vi "H5D Create 1D array.vi"(5 "chunk size":u32=16250, 6 "compress level":i32=9, 7 "compress?":bool, 8 "error in (no error)":errorcluster, 9 "defined type":i32(ring)=17 items=["None", "IEEE_F32BE", "IEEE_F32LE", "IEEE_F64BE", "IEEE_F64LE", "NATIVE_CHAR", "NATIVE_SCHAR", "NATIVE_UCHAR", "NATIVE_SHORT", "NATIVE_USHORT", "NATIVE_INT", "NATIVE_UINT", "NATIVE_LONG", "NATIVE_ULONG", "NATIVE_LLONG", "NATIVE_ULLONG", "NATIVE_FLOAT", "NATIVE_DOUBLE", "NATIVE_LDOUBLE", "NATIVE_B8", "NATIVE_B16", "NATIVE_B32", "NATIVE_B64", "NATIVE_OPAQUE", "NATIVE_HADDR", "NATIVE_HSIZE", "NATIVE_HSSIZE", "NATIVE_HERR", "NATIVE_HBOOL", "STD_U8LE", "STD_U8BE", "STD_U16LE", "STD_U16BE", "STD_U32LE", "STD_U32BE", "STD_U64LE", "STD_U64BE", "STD_B8LE", "STD_B8BE", "STD_B16LE", "STD_B16BE", "STD_B32LE", "STD_B32BE", "STD_B64LE", "STD_B64BE", "STD_REF_OBJ", "STD_REF_DSETREG", "C_S1", "STD_I8LE", "STD_I8BE", "STD_I16LE", "STD_I16BE", "STD_I32LE", "STD_I32BE", "STD_I64LE", "STD_I64BE", ""], 10 "name":string, 11 "loc_id":i32) -> (0 "error out":errorcluster, 1 "space_id":i32, 2 "plist out":i32, 3 "dataset_id":i32)   [LabVIEW 2011]
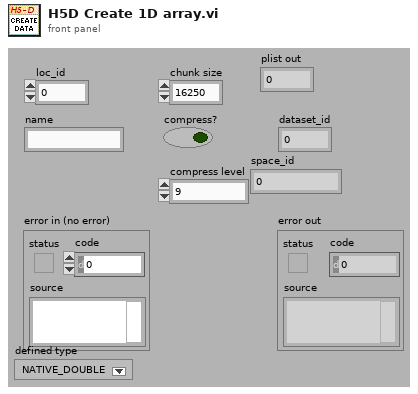
[diagram p1: front panel]
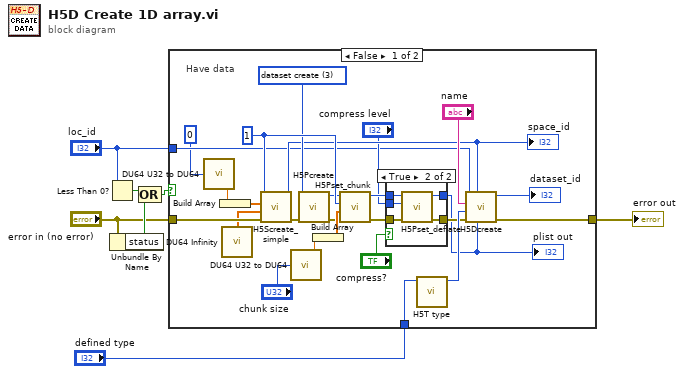
[diagram p0: block diagram]
diagram:
  n1 = Less Than 0?(x="loc_id") -> (x < 0?=w5:bool)
  n2 = Unbundle By Name("error in (no error)") -> ("status"=w6:bool)
  n3 = Compound Arithmetic op=OR(w5, w6) -> (w4:bool)
  n4 = case shown="False" w4 {
    tunnel: [w12 w41] -> w7
    tunnel: "error in (no error)" -> [w23 w41]
    tunnel: "loc_id" -> [w15 _]
    tunnel: "defined type" -> [w13 _]
    frame False {
      w31 = 1 ("rank")
      w27 = 3 items=["no class", "file create", "file access", "dataset create", "dataset transfer", "mount", "n classes"] ("pclass")
      # "Have data"
      n5 = call <instrlib>:"DU64 U32 to DU64.vi"("U32"=u32 0) -> ("DU64"=w9:dbl)
      n6 = Build Array(w9) -> (w25:dbl[])
      n7 = call <instrlib>:"DU64 Infinity.vi"() -> ("DU64 maxdims"=w10:dbl[])
      n8 = call <instrlib>:"H5Screate_simple.vi"("error in (no error)"=w23, "DU64 maxdims"=w10, "DU64 dims"=w25, "rank"=w31) -> ("error out"=w29:errorcluster, "space_id"=w24:i32)  [unwired: 6 in]
      "space_id" <- w24
      n9 = call <instrlib>:"DU64 U32 to DU64.vi"("U32"="chunk size") -> ("DU64"=w17:dbl)
      n10 = call <instrlib>:"H5Pcreate.vi"("error in (no error)"=w29, "pclass"=w27) -> ("error out"=w28:errorcluster, "plist"=w30:i32)  [unwired: 8 in]
      n11 = Build Array(w17) -> (w32:dbl[])
      n12 = call <instrlib>:"H5Pset_chunk.vi"("error in (no error)"=w28, "DU64 dim"=w32, "ndims"=w31, "plist in"=w30) -> ("error out"=w22:errorcluster, "plist out"=w21:i32)  [unwired: 6 in]
      n13 = case shown="True" "compress?" {
        tunnel: w22 -> [w34 w40]
        tunnel: w21 -> [w35 w39]
        tunnel: [w35 w38] -> w14
        tunnel: [w34 w37] -> w20
        tunnel: "compress level" -> [_ w36]
        frame False {
        }
        frame True {
          n14 = call <instrlib>:"H5Pset_deflate.vi"("error in (no error)"=w40, "level"=w36, "plist in"=w39) -> ("error out"=w37:errorcluster, "plist out"=w38:i32)  [unwired: 7 in]
        }
      }
      "plist out" <- w14
      n15 = call <instrlib>:"H5T type.vi"("defined type"=w13) -> ("type_id"=w26:i32)  [unwired: 10 in]
      n16 = call <instrlib>:"H5Dcreate.vi"("create_plist_id"=w14, "space_id"=w24, "error in (no error)"=w20, "type_id"=w26, "name"="name", "loc_id"=w15) -> ("error out"=w12:errorcluster, "dataset_id"=→"dataset_id":i32)  [unwired: 4 in]
    }
    frame True {
      # "No data or error"
    }
  }
  "error out" <- w7
